vi "Write Test Names.vi"(8 "error in (no error)":errorcluster, 10 "Test Names":string[](array[string]), 11 "Test Selector in":refnum<class "Test Selector.lvclass">) -> (0 "error out":errorcluster, 3 "Test Selector out":refnum<class "Test Selector.lvclass">)   [LabVIEW 2019, in "Test Selector.lvlib" / "Test Selector.lvclass"]
uses:
  Test Selector.lvclass
  Test Selector.lvclass/Test Selector.ctl
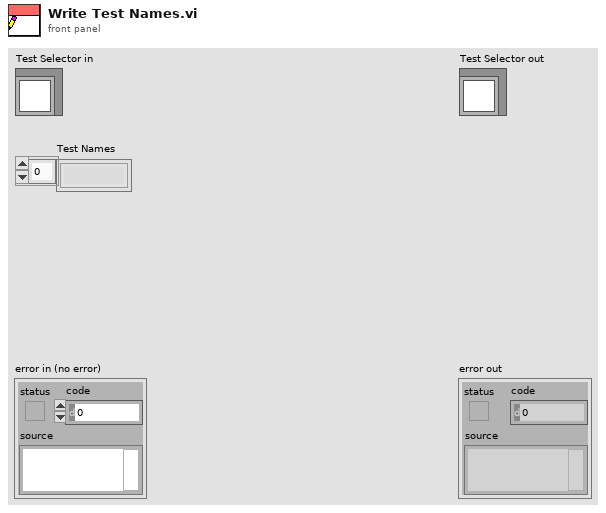
[diagram p1: front panel]
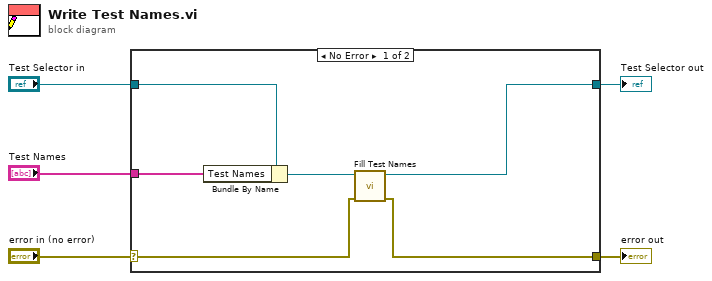
[diagram p0: block diagram]
diagram:
  n1 = case shown="No Error" "error in (no error)" {
    selector: "error in (no error)" -> [w8 w12]
    tunnel: [w6 w12] -> w4
    tunnel: [w7 w13] -> w2
    tunnel: "Test Selector in" -> [w11 w13]
    tunnel: "Test Names" -> [w10 _]
    frame No Error {
      n2 = Bundle By Name(cluster=w11, "Test Names"=w10) -> (w9:refnum<class "Test Selector.lvclass">)
      n3 = call "Fill Test Names.vi"("error in (no error)"=w8, "Test Selector in"=w9) -> ("error out"=w6:errorcluster, "Test Selector out"=w7:refnum<class "Test Selector.lvclass">)  [unwired: 8 in]
    }
    frame Error {
    }
  }
  "error out" <- w4
  "Test Selector out" <- w2
